vi "Perform Self Test.vi"(6 "Wait for Reply?":bool=TRUE, 8 "error in (no error)":errorcluster, 11 "Device Under Test In":refnum<class "Device Under Test.lvclass">) -> (0 "error out":errorcluster, 1 "Timed out?":bool, 2 "data":T1, 3 "Device Under Test Out":refnum<class "Device Under Test.lvclass">)   [LabVIEW 2020, in "Device Under Test.lvclass"]
uses:
  Device Under Test.lvclass
  C:/Program Files (x86)/National Instruments/LabVIEW 2020/vi.lib/Astemes/Triarc Framework/Process/Process.lvclass
  Private/Self Test Reply Payload.ctl
  <vilib>/Astemes/Triarc Framework/Process/Process.lvclass/Process.ctl
  <vilib>/Astemes/Triarc Framework/Process/Public/Lifecycle/Get Lifecycle State.vi
  <vilib>/Astemes/Triarc Framework/Process/Private/SubVIs/Handle Debug Data.vi
  <vilib>/Astemes/Triarc Framework/Process/Private/SubVIs/Enqueue Request Message.vi
  <vilib>/Utility/error.llb/Clear Errors.vi
  <vilib>/Utility/High Resolution Relative Seconds.vi
  <vilib>/Utility/error.llb/Error Cluster From Error Code.vi
  <vilib>/Astemes/Triarc Framework/Process/Private/SubVIs/Wait for Response Message.vi
  <vilib>/Astemes/Triarc Framework/Process/Process.lvclass
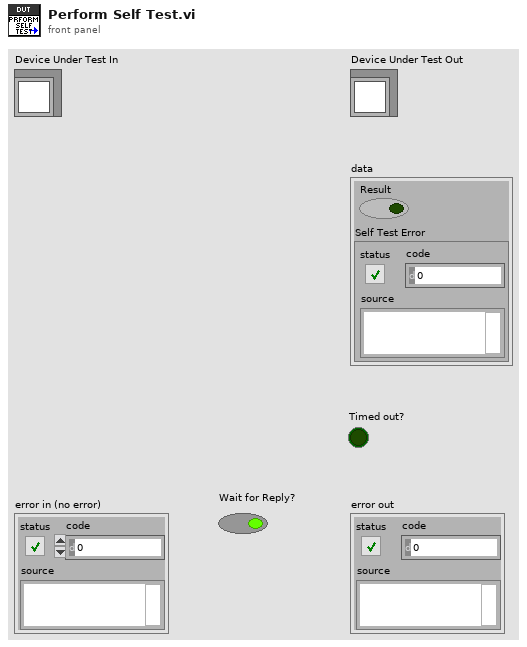
[diagram p1: front panel]
types:
  T1 = typedef "Device Under Test.lvclass/Self Test Reply Payload.ctl" = cluster{"Result":bool, "Self Test Error":errorcluster}
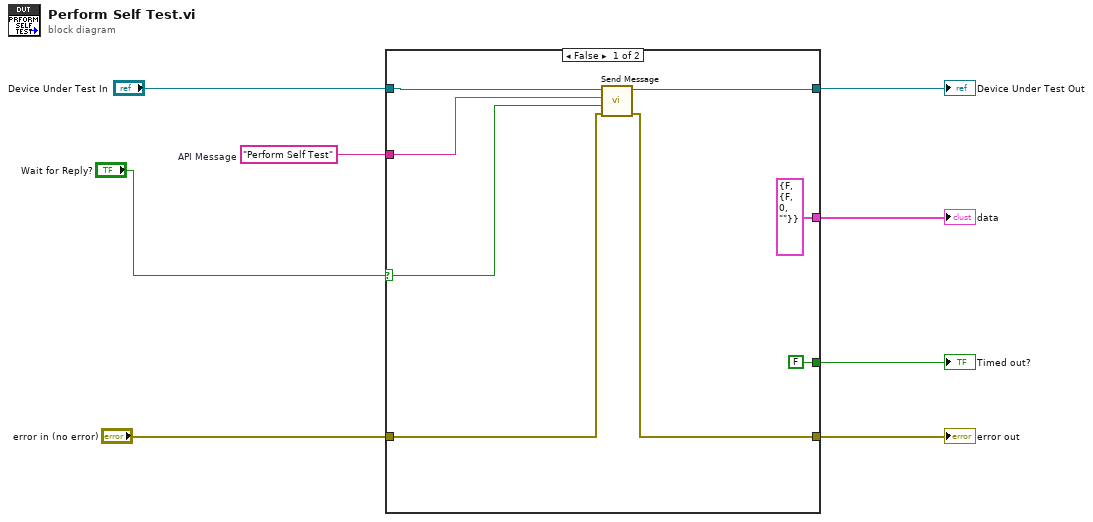
[diagram p0: block diagram]
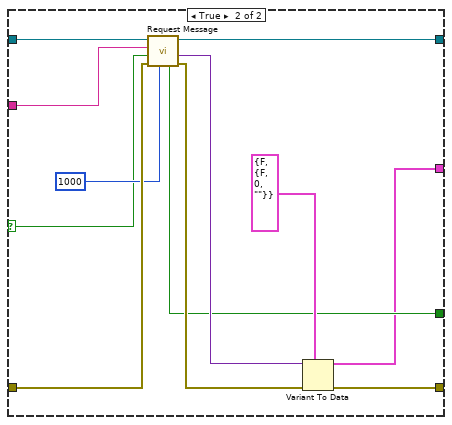
[diagram p2: hidden frame]
diagram:
  w6 = "Perform Self Test"  # API Message
  n1 = case shown="False" "Wait for Reply?" {
    selector: "Wait for Reply?" -> [w9 w17]
    tunnel: [w14 w28] -> w8
    tunnel: "error in (no error)" -> [w13 w26]
    tunnel: w6 -> [w15 w25]
    tunnel: "Device Under Test In" -> [w16 w24]
    tunnel: [w12 w22] -> w4
    tunnel: [FALSE ("Timed out?") w19] -> w3
    tunnel: [T1 {"Result"=FALSE, "Self Test Error"={"status"=FALSE, "code"=0, "source"=""}} ("Perform Self Test (Reply Payload)") w18] -> w2
    frame False {
      n2 = call <vilib>:"Send Message.vi"("error in (no error)"=w13, "Message Data"=w9, "Message"=w15, "Process In"=w16) -> ("error out"=w12:errorcluster, "Process Out"=w14:refnum<class "Device Under Test.lvclass">)  [unwired: 6 in]
    }
    frame True {
      n3 = call <vilib>:"Request Message.vi"("timeout in ms (-1)"=1000, "error in (no error)"=w26, "Request Message Data"=w17, "Request Message"=w25, "Process In"=w24) -> ("error out"=w27:errorcluster, "Response Message Data"=w20:variant, "Process Out"=w28:refnum<class "Device Under Test.lvclass">, "Timed out?"=w19:bool)  [unwired: 2 in, 1 out]
      n4 = Variant To Data(error in=w27, type=T1 {"Result"=FALSE, "Self Test Error"={"status"=FALSE, "code"=0, "source"=""}} ("Perform Self Test (Reply Payload)"), Variant=w20) -> (data=w18:T1, error out=w22:errorcluster)
    }
  }
  "error out" <- w4
  "Device Under Test Out" <- w8
  "Timed out?" <- w3
  "data" <- w2
